vi "Configure CMOS.vi"() -> ()   [LabVIEW 2013, in "Stanford Research CG635.lvlib"]
uses:
  <instrlib>/Stanford Research CG635/Stanford Research CG635.lvlib
panel:
  in  "CMOS High (5 V)":dbl=5.0
  in  "CMOS Low (0 V)":dbl
  out "VISA resource name out":refnum<visa-resource-name>
  out "error out":errorcluster
  in  "VISA resource name":refnum<visa-resource-name>
  in  "error in (no error)":errorcluster
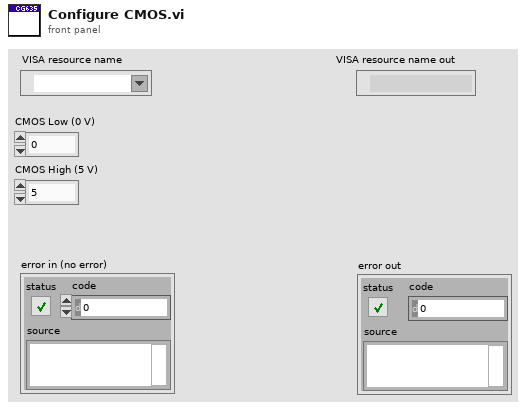
[diagram p1: front panel]
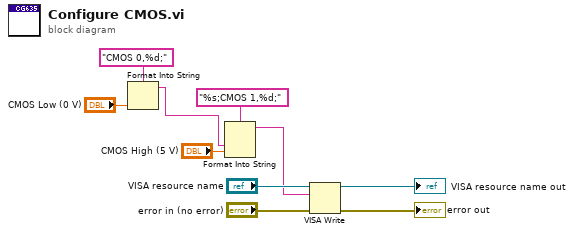
[diagram p0: block diagram]
diagram:
  n1 = Format Into String(format string="CMOS 0,%d;", "CMOS Low (0 V)") -> (resulting string=w2:string)  [unwired: 2 in, 1 out]
  n2 = Format Into String(format string="%s;CMOS 1,%d;", w2, "CMOS High (5 V)") -> (resulting string=w1:string)  [unwired: 2 in, 1 out]
  n3 = VISA Write(VISA resource name="VISA resource name", write buffer=w1, error in (no error)="error in (no error)") -> (VISA resource name out=→"VISA resource name out":refnum<visa-resource-name>, error out=→"error out":errorcluster)  [unwired: 1 out]
